vi "axex_rename_sheet.vi"(8 "error in":errorcluster, 10 "new name":string, 11 "AX Excel instance in":T1) -> (0 "error out":errorcluster, 3 "AX Excel instance out":T1)   [LabVIEW 2020, in "AX Excel.lvlib"]
doc: "Call this to rename current sheet."
uses:
  AX Excel.lvlib
  axex_instance.ctl
  <vilib>/Utility/error.llb/Error Cluster From Error Code.vi
  <vilib>/ErrorRing/Error Ring.xnode
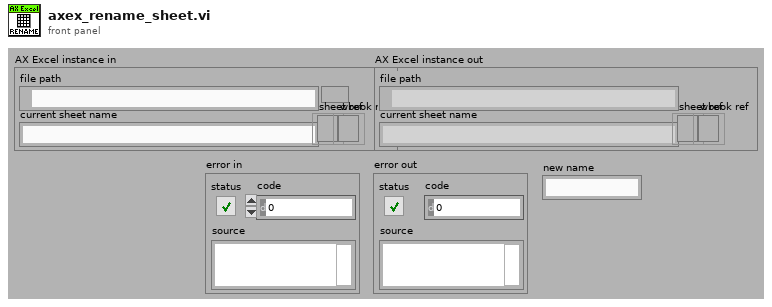
[diagram p1: front panel]
types:
  T1 = typedef "AX Excel.lvlib/axex_instance.ctl" = cluster{"file path":path, "current sheet name":string, "sheet ref":refnum<k7>, "wbook ref":refnum<k7>}
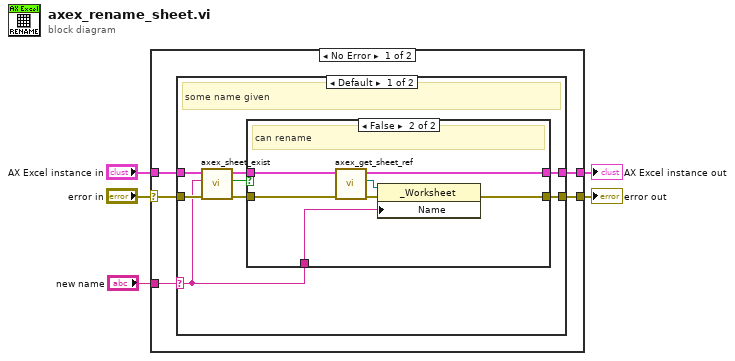
[diagram p0: block diagram]
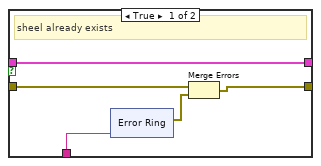
[diagram p2: hidden frame]
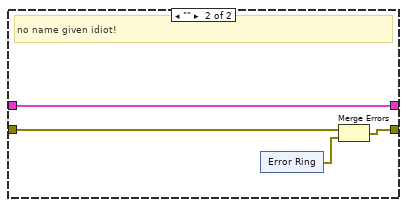
[diagram p3: hidden frame]
diagram:
  n1 = case shown="No Error" "error in" {
    selector: "error in" -> [w6 w48]
    tunnel: "new name" -> [w10 _]
    tunnel: "AX Excel instance in" -> [w9 w47]
    tunnel: [w8 w48] -> w3
    tunnel: [w7 w47] -> w2
    frame No Error {
      n2 = case shown="Default" w10 {
        selector: w10 -> [w14 _]
        tunnel: w6 -> [w16 w40]
        tunnel: w9 -> [w15 w38]
        tunnel: [w17 w39] -> w8
        tunnel: [w18 w38] -> w7
        frame Default {
          # "some name given"
          n3 = call "axex_sheet_exist.vi"("error in"=w16, "sheet name"=w14, "AX Excel instance in"=w15) -> ("error out"=w12:errorcluster, "sheet found?"=w13:bool, "AX Excel instance out"=w11:T1)  [unwired: 3 in, 3 out]
          n4 = case shown="False" w13 {
            tunnel: [w19 w37] -> w18
            tunnel: [w21 w34] -> w17
            tunnel: w14 -> [w20 w33]
            tunnel: w12 -> [w22 w32]
            tunnel: w11 -> [w19 w31]
            frame True {
              # "sheel already exists"
              n5 = xnode "Error Ring"("parameter 0"=w20) -> ("error out"=w23:errorcluster)
              n6 = Merge Errors(w22, w23) -> (w21:errorcluster)
            }
            frame False {
              # "can rename"
              n7 = call "axex_get_sheet_ref.vi"("error in"=w32, "AX Excel instance in"=w31) -> ("error out"=w36:errorcluster, "sheet ref out"=w35:refnum<k7>, "AX Excel instance out"=w37:T1)  [unwired: 6 in, 1 out]
              n8 = property class="_Worksheet"(reference=w35, error in=w36, "Name"=w33) -> (error out=w34:errorcluster)  [unwired: 1 out]
            }
          }
        }
        frame "" {
          # "no name given idiot!"
          n9 = xnode "Error Ring"() -> ("error out"=w41:errorcluster)
          n10 = Merge Errors(w40, w41) -> (w39:errorcluster)
        }
      }
    }
    frame Error {
    }
  }
  "error out" <- w3
  "AX Excel instance out" <- w2
